vi "Raw_BG_correction.vi"(7 "Change?":bool, 8 "error in (no error)":errorcluster, 10 "raw bg":i32[](array[numeric]), 11 "Control-Client in":refnum<class "Control-Client.lvclass">) -> (0 "error out":errorcluster, 3 "Control-Client out":refnum<class "Control-Client.lvclass">)   [LabVIEW 2018, in "Control-Client.lvclass"]
uses:
  Control-Client.lvclass
  Control-Client.lvclass/Control-Client.ctl
  Experiments/Experiment.lvclass
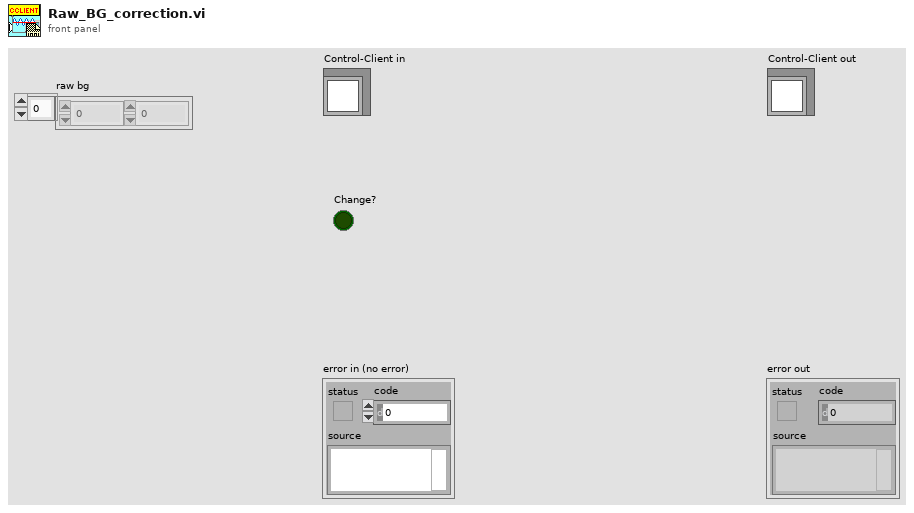
[diagram p1: front panel]
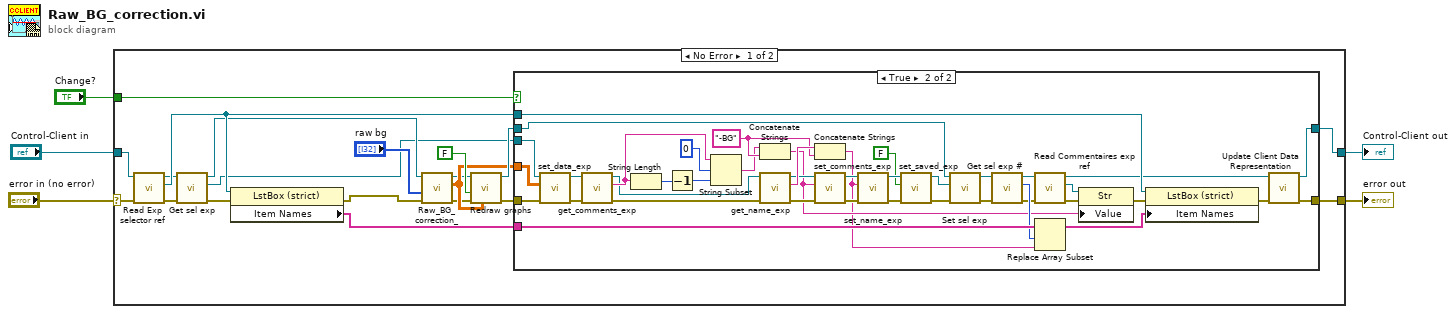
[diagram p0: block diagram]
diagram:
  n1 = case shown="No Error" "error in (no error)" {
    selector: "error in (no error)" -> [w25 w70]
    tunnel: [w20 w70] -> w4
    tunnel: [w19 w69] -> w2
    tunnel: "Control-Client in" -> [w24 w69]
    tunnel: "Change?" -> [w13 _]
    frame No Error {
      n2 = call "Read Exp selector ref.vi"("error in (no error)"=w25, "Control-Client in"=w24) -> ("error out"=w16:errorcluster, "Exp selector ref"=w22:refnum<vi>, "Control-Client out"=w17:refnum<class "Control-Client.lvclass">)  [unwired: 7 in]
      n3 = call "Get sel exp.vi"("error in (no error)"=w16, "Control-Client in"=w17) -> ("error out"=w21:errorcluster, "Sel experiment"=w7:refnum<class "Experiment.lvclass">, "Control-Client out"=w10:refnum<class "Control-Client.lvclass">)  [unwired: 7 in]
      n4 = property on="Property Node" class="LstBox (strict)"(reference=w22, error in=w21) -> (error out=w6:errorcluster, "Item Names"=w23:string[])  [unwired: 1 out]
      n5 = call "Raw_BG_correction_.vi"("error in (no error)"=w6, "raw bg"="raw bg", "Control-Client en entrée"=w10) -> ("error out"=w8:errorcluster, "Data corrected"=w12:dbl[][], "Control-Client en sortie"=w9:refnum<class "Control-Client.lvclass">)  [unwired: 6 in]
      n6 = call "Redraw graphs.vi"("Data"=w12, "error in (no error)"=w8, "Selected exp"=FALSE, "Control-Client in"=w9) -> ("error out"=w15:errorcluster, "Control-Client out"=w14:refnum<class "Control-Client.lvclass">)  [unwired: 6 in]
      n7 = case shown="True" w13 {
        tunnel: w23 -> [_ w68]
        tunnel: w22 -> [_ w67]
        tunnel: [w26 w66] -> w20
        tunnel: [w27 w65] -> w19
        tunnel: w12 -> [_ w35]
        tunnel: w15 -> [w26 w30]
        tunnel: w7 -> [_ w29]
        tunnel: w14 -> [w27 w28]
        frame False {
        }
        frame True {
          w57 = "-BG" ("string")
          n8 = call "set_data_exp.vi"("error in (no error)"=w30, "Data"=w35, "Experiment.lvclass in"=w29) -> ("error out"=w41:errorcluster, "Experiment.lvclass out"=w42:refnum<class "Experiment.lvclass">)  [unwired: 7 in]
          n9 = call "get_comments_exp.vi"("error in (no error)"=w41, "Experiment.lvclass in"=w42) -> ("error out"=w63:errorcluster, "Comments"=w55:string, "Experiment.lvclass out"=w44:refnum<class "Experiment.lvclass">)  [unwired: 7 in]
          n10 = String Length(string=w55) -> (length=w53:i32)
          n11 = Decrement(x=w53) -> (x-1=w52:i32)
          n12 = String Subset(string=w55, offset (0)=0, length (rest)=w52) -> (substring=w51:string)
          n13 = Concatenate Strings(w51, w57) -> (w34:string)
          n14 = call "get_name_exp.vi"("error in (no error)"=w63, "Experiment.lvclass in"=w44) -> ("error out"=w64:errorcluster, "Exp name"=w62:string, "Experiment.lvclass out"=w43:refnum<class "Experiment.lvclass">)  [unwired: 7 in]
          n15 = Concatenate Strings(w62, w57) -> (w33:string)
          n16 = call "set_comments_exp.vi"("error in (no error)"=w64, "Comments"=w34, "Experiment.lvclass in"=w43) -> ("error out"=w60:errorcluster, "Experiment.lvclass out"=w61:refnum<class "Experiment.lvclass">)  [unwired: 7 in]
          n17 = call "set_name_exp.vi"("error in (no error)"=w60, "Exp name"=w33, "Experiment.lvclass in"=w61) -> ("error out"=w58:errorcluster, "Experiment.lvclass out"=w59:refnum<class "Experiment.lvclass">)  [unwired: 7 in]
          n18 = call "set_saved_exp.vi"("error in (no error)"=w58, "Saved"=FALSE, "Experiment.lvclass in"=w59) -> ("error out"=w31:errorcluster, "Experiment.lvclass out"=w32:refnum<class "Experiment.lvclass">)  [unwired: 7 in]
          n19 = call "Set sel exp.vi"("error in (no error)"=w31, "Experiment"=w32, "Control-Client in"=w28) -> ("error out"=w38:errorcluster, "Control-Client out"=w45:refnum<class "Control-Client.lvclass">)  [unwired: 7 in]
          n20 = call "Get sel exp #.vi"("error in (no error)"=w38, "Control-Client in"=w45) -> ("error out"=w37:errorcluster, "Exp sel #"=w49:i32, "Control-Client out"=w40:refnum<class "Control-Client.lvclass">)  [unwired: 7 in]
          n21 = call "Read Commentaires exp ref.vi"("error in (no error)"=w37, "Control-Client in"=w40) -> ("error out"=w47:errorcluster, "Commentaires exp ref"=w48:refnum<vi>, "Control-Client out"=w39:refnum<class "Control-Client.lvclass">)  [unwired: 7 in]
          n22 = Replace Array Subset(array=w68, new element=w33, index=w49) -> (w50:string[])
          n23 = property on="Property Node" class="Str"(reference=w48, error in=w47, "Value"=w34) -> (error out=w46:errorcluster)  [unwired: 1 out]
          n24 = property on="Property Node" class="LstBox (strict)"(reference=w67, error in=w46, "Item Names"=w50) -> (error out=w36:errorcluster)  [unwired: 1 out]
          n25 = call "Update Client Data Representation.vi"("error in (no error)"=w36, "Control-Client in"=w39) -> ("error out"=w66:errorcluster, "Control-Client out"=w65:refnum<class "Control-Client.lvclass">)  [unwired: 8 in]
        }
      }
    }
    frame Error {
    }
  }
  "error out" <- w4
  "Control-Client out" <- w2
